vi "ISO-8601 Format Strings.vi"() -> (1 "Formats":string[][][](array[string])=[[["%^<%Y-%m-%dT%H:%M:%S%3uZ>T", "%^<%Y%m%dT%H%M%S%3uZ>T"], ["%^<%Y-%m-%dT%H:%M:%SZ>T", "%^<%Y%m%dT%H%M%SZ>T"], ["%^<%Y-%m-%dT%H:%MZ>T", "%^<%Y%m%dT%H%MZ>T"], ["%^<%Y-%m-%dT%HZ>T", "%^<%Y%m%dT%HZ>T"], ["%^<%Y-%m-%dZ>T", "%^<%Y%m%dZ>T"]]])   [LabVIEW 2020, in "CDM-Config.lvlib"]
uses:
  CDM-Config.lvlib
  Precision.ctl
  Format.ctl
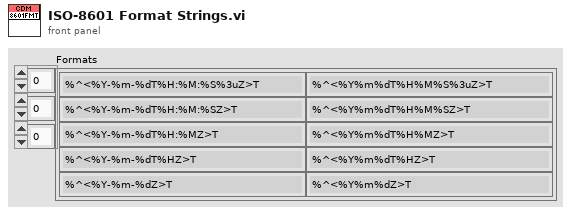
[diagram p1: front panel]
types:
  T1 = typedef "CDM-Config.lvlib/Format.ctl" = enum16{"Extended", "Basic"}
  T2 = typedef "CDM-Config.lvlib/Precision.ctl" = enum16{"Millisecond", "Second", "Minute", "Hour", "Day"}
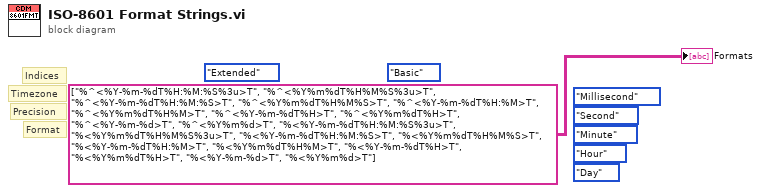
[diagram p0: block diagram]
diagram:
  (unwired) Format."Basic" ("Format")
  (unwired) Format."Extended" ("Format")
  (unwired) Precision."Day" ("Precision")
  (unwired) Precision."Hour" ("Precision")
  (unwired) Precision."Minute" ("Precision")
  (unwired) Precision."Millisecond" ("Precision")
  (unwired) Precision."Second" ("Precision")
  # "Timezone"
  # "Indices"
  # "Format"
  # "Precision"
  "Formats" <- string[][][] [[["%^<%Y-%m-%dT%H:%M:%S%3u>T", "%^<%Y%m%dT%H%M%S%3u>T"], ["%^<%Y-%m-%dT%H:%M:%S>T", "%^<%Y%m%dT%H%M%S>T"], ["%^<%Y-%m-%dT%H:%M>T", "%^<%Y%m%dT%H%M>T"], ["%^<%Y-%m-%dT%H>T", "%^<%Y%m%dT%H>T"], ["%^<%Y-%m-%d>T", "%^<%Y%m%d>T"]], [["%<%Y-%m-%dT%H:%M:%S%3u>T", "%<%Y%m%dT%H%M%S%3u>T"], ["%<%Y-%m-%dT%H:%M:%S>T", "%<%Y%m%dT%H%M%S>T"], ["%<%Y-%m-%dT%H:%M>T", "%<%Y%m%dT%H%M>T"], ["%<%Y-%m-%dT%H>T", "%<%Y%m%dT%H>T"], ["%<%Y-%m-%d>T", "%<%Y%m%d>T"]]]
